vi "updateList.vi"(8 "error in (no error)":errorcluster, 10 "Listbox":refnum<vi>, 11 "ExperimentRunner in":refnum<class "ExperimentRunner.lvclass">) -> (0 "error out":errorcluster, 2 "Listbox out":refnum<vi>, 3 "ExperimentRunner out":refnum<class "ExperimentRunner.lvclass">)   [LabVIEW 2009, in "Views.lvlib" / "ExperimentControl.lvlib" / "ExperimentRunner.lvclass"]
doc: "Adds the new Script path name to the Front End."
uses:
  ExperimentRunner.lvclass
  ExperimentRunner.lvclass/ExperimentRunner.ctl
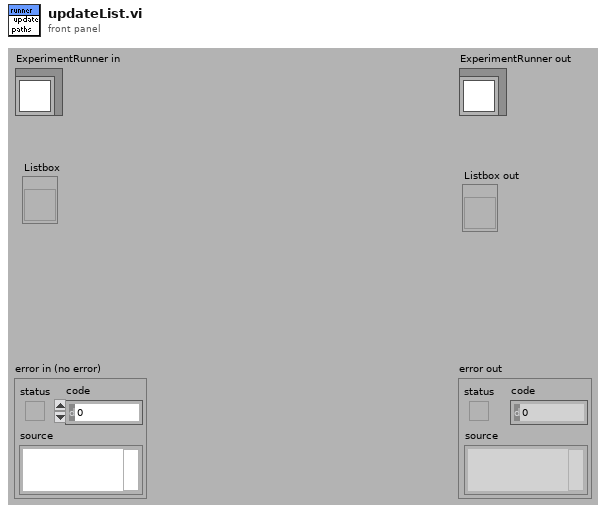
[diagram p1: front panel]
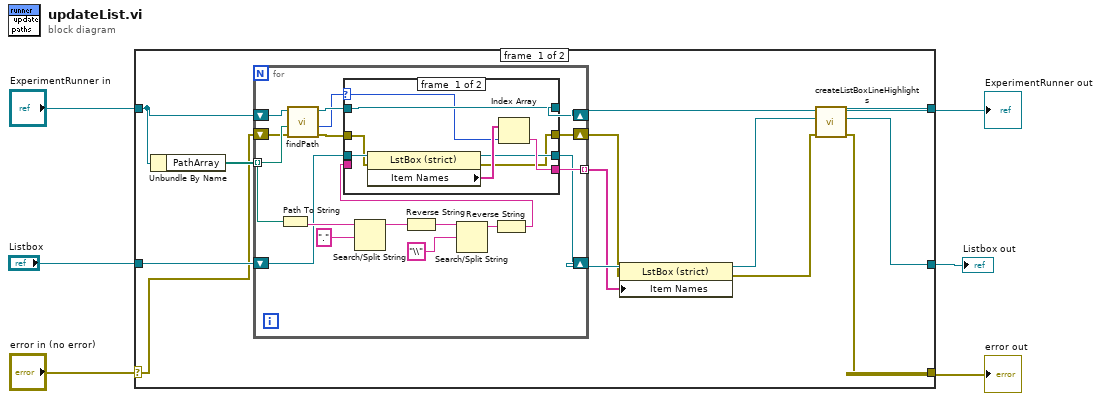
[diagram p0: block diagram]
diagram:
  n1 = case shown="No Error" "error in (no error)" {
    selector: "error in (no error)" -> [w8 w51]
    tunnel: [w14 w51] -> w5
    tunnel: [w13 w50] -> w3
    tunnel: "ExperimentRunner in" -> [w10 w50]
    tunnel: "Listbox" -> [w18 _]
    tunnel: [w11 _] -> w1
    frame #0 {
      n2 = Unbundle By Name(w10) -> ("PathArray"=w19:path[])
      n3 = for {
        tunnel: w19 -> [w30] mode=indexing
        tunnel: [w26] -> w16 mode=indexing
        shift-right: [w23] -> w17
        shift-left: w18 -> [w24]
        shift-right: [w25] -> w9
        shift-left: w10 -> [w31]
        shift-right: [w20] -> w7
        shift-left: w8 -> [w22]
        n4 = Path To String(path=w30) -> (string=w37:string)
        n5 = call "findPath.vi"("error in (no error)"=w22, "Path"=w30, "ExperimentRunner in"=w31) -> ("error out"=w21:errorcluster, "index of element"=w28:i32, "ExperimentRunner out"=w29:refnum<class "ExperimentRunner.lvclass">)  [unwired: 6 in]
        n6 = Search/Split String(string=w37, search string/char (-)=".") -> (substring before match=w35:string)  [unwired: 1 in, 2 out]
        n7 = Reverse String(1:w35) -> (0:w34:string)
        n8 = Search/Split String(string=w34, search string/char (-)="\\") -> (substring before match=w32:string)  [unwired: 1 in, 2 out]
        n9 = Reverse String(1:w32) -> (0:w27:string)
        n10 = case shown="0, Default" w28 {
          selector: w28 -> [w42 _]
          tunnel: w29 -> [w45 w48]
          tunnel: w27 -> [_ w49]
          tunnel: [w41 w49] -> w26
          tunnel: [w45 w48] -> w25
          tunnel: w24 -> [w44 w47]
          tunnel: [w40 w47] -> w23
          tunnel: w21 -> [w39 w46]
          tunnel: [w38 w46] -> w20
          frame #0 {
            n11 = property class="LstBox (strict)"(reference=w44, error in=w39) -> (reference out=w40:refnum<vi>, error out=w38:errorcluster, "Item Names"=w43:string[])
            n12 = Index Array(array=w43, index=w42) -> (element=w41:string)
          }
          frame #1 {
          }
        }
      }
      n13 = property class="LstBox (strict)"(reference=w17, error in=w7, "Item Names"=w16) -> (reference out=w12:refnum<vi>, error out=w15:errorcluster)
      n14 = call "createListBoxLineHighlights.vi"("error in (no error)"=w15, "Listbox in"=w12, "ExperimentRunner in"=w9) -> ("error out"=w14:errorcluster, "Listbox out"=w11:refnum<vi>, "ExperimentRunner out"=w13:refnum<class "ExperimentRunner.lvclass">)  [unwired: 6 in]
    }
    frame #1 {
    }
  }
  "error out" <- w5
  "ExperimentRunner out" <- w3
  "Listbox out" <- w1
